vi "dotted.vi"(7 "N times":i32, 8 "error in (no error)":errorcluster, 9 "Time Dots (ms)":u32, 10 "Space bet dots (mm)":dbl, 11 "VISA Refnum in":refnum<visa-resource-name>) -> (0 "error out":errorcluster, 3 "VISA Refnum out":refnum<visa-resource-name>)   [LabVIEW 2014]
doc: "Newport Motion Controler\nThis sub program make dots structure\n\nAndré Romero - 2022\nandretec@ifsc.usp.br"
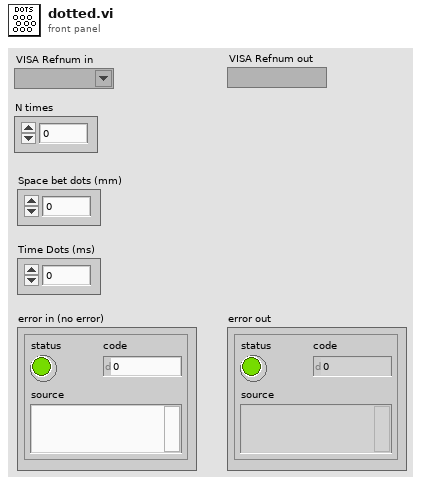
[diagram p1: front panel]
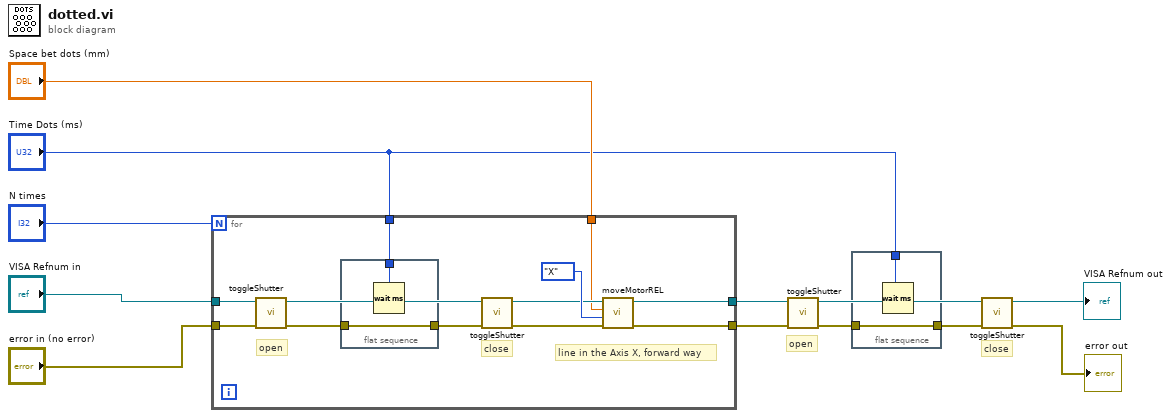
[diagram p0: block diagram]
diagram:
  # "close"
  # "open"
  n1 = for {
    N: "N times" -> [_]
    tunnel: "VISA Refnum in" -> [w17]
    tunnel: [w19] -> w3
    tunnel: "error in (no error)" -> [w16]
    tunnel: [w18] -> w4
    tunnel: "Space bet dots (mm)" -> [w12]
    tunnel: "Time Dots (ms)" -> [w11]
    # "close"
    # "open"
    # "line in the Axis X, forward way"
    n2 = call "toggleShutter.vi"("Error In"=w16) -> ("error out"=w15:errorcluster)  [unwired: 9 in]
    n3 = flat-sequence {
      tunnel: w15 -> [w22]
      tunnel: [w22] -> w14
      tunnel: w11 -> [w21]
      frame #0 {
        n4 = Wait (ms)(milliseconds to wait=w21) -> ()  [unwired: 1 out]
      }
    }
    n5 = call "toggleShutter.vi"("Error In"=w14) -> ("error out"=w13:errorcluster)  [unwired: 9 in]
    n6 = call "moveMotorREL.vi"("error in (no error)"=w13, "Axis"=enum16{"X", "Y"}."X", "L (mm)"=w12, "VISA Refnum in"=w17) -> ("error out"=w18:errorcluster, "VISA Refnum out"=w19:refnum<visa-resource-name>)  [unwired: 6 in]
  }
  "VISA Refnum out" <- w3
  n7 = call "toggleShutter.vi"("Error In"=w4) -> ("error out"=w6:errorcluster)  [unwired: 9 in]
  n8 = flat-sequence {
    tunnel: w6 -> [w24]
    tunnel: [w24] -> w5
    tunnel: "Time Dots (ms)" -> [w23]
    frame #0 {
      n9 = Wait (ms)(milliseconds to wait=w23) -> ()  [unwired: 1 out]
    }
  }
  n10 = call "toggleShutter.vi"("Error In"=w5) -> ("error out"=→"error out":errorcluster)  [unwired: 9 in]
